vi "Busqueda en diagrama de bloques.vi"   [LabVIEW 2020]
uses:
  <vilib>/Utility/traverseref.llb/TRef TravTarget.ctl
  <vilib>/Utility/traverseref.llb/VI Scripting - Traverse.lvlib
types:
  T1 = typedef "TRef TravTarget.ctl" = enum16{"FP", "BD", "Other"}
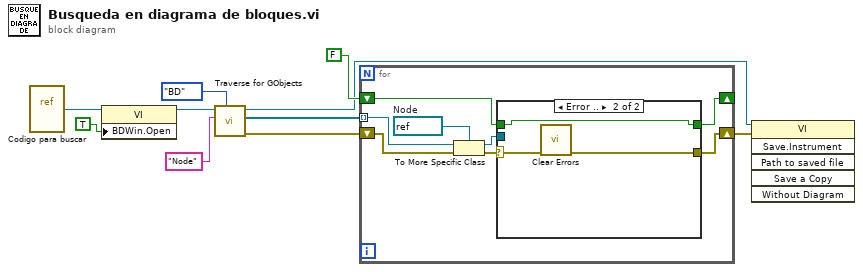
[diagram p0: block diagram]
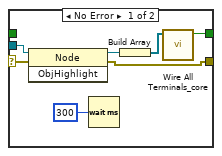
[diagram p2: hidden frame]
diagram:
  n1 = vi-ref "Codigo para buscar.vi"() -> (w9:refnum<vi>)
  n2 = property class="VI"(reference=w9, "BDWin.Open"=TRUE ("Block Diagram Window:Open")) -> (reference out=w6:refnum<vi>)  [unwired: 1 in, 1 out]
  n3 = call <vilib>:"Traverse for GObjects.vi"("Traverse Target"=TRef_TravTarget."BD", "Class Name"="Node", "VI Refnum"=w6) -> ("error out"=w10:errorcluster, "References"=w3:refnum<vi>[], "dup VI Refnum"=w2:refnum<vi>)  [unwired: 5 in, 1 out]
  n4 = for {
    tunnel: w3 -> [w16] mode=indexing
    shift-right: [w13] -> _
    shift-left: FALSE ("changes made?") -> [w12]
    shift-right: [w11] -> w1
    shift-left: w10 -> [w18]
    w15 = refnum<vi> refnum  # Node
    n5 = To More Specific Class(target class=w15, reference=w16, error in=w18) -> (specific class reference=w14:refnum<vi>, error out=w17:errorcluster)
    n6 = case shown="Error .." w17 {
      selector: w17 -> [w25 w27]
      tunnel: w14 -> [w24 _]
      tunnel: [w20 w28] -> w13
      tunnel: w12 -> [_ w28]
      tunnel: [w19 w26] -> w11
      frame No Error {
        n7 = invoke class="Node" method="ObjHighlight"(reference=w24, error in=w25) -> (reference out=w22:refnum<vi>, error out=w19:errorcluster)  [unwired: 1 in, 1 out]
        n8 = Wait (ms)(milliseconds to wait=u32 300) -> ()  [unwired: 1 out]
        n9 = Build Array(w22) -> (w21:refnum<vi>[])
        n10 = call <vilib>:"Wire All Terminals_core.vi"("SelList[]"=w21) -> ("changes made?"=w20:bool)  [unwired: 9 in, 1 out]
      }
      frame Error {
        n11 = call <vilib>:"Clear Errors.vi"("error in (no error)"=w27) -> ("error out"=w26:errorcluster)  [unwired: 5 in, 1 out]
      }
    }
  }
  n12 = invoke class="VI" method="Save.Instrument"(reference=w2, error in=w1) -> ()  [unwired: 4 in, 6 out]
